vi "Initialize - Packet Page Panel.vi"(7 "Channels Listbox":refnum<vi>, 8 "error in (no error)":errorcluster, 11 "Item Ref in":T1 format="%.0x") -> (0 "error out":errorcluster, 3 "Item Ref out":T1 format="%.0x")   [LabVIEW 2019, in "UDP-Custom-Device System Explorer.lvlib"]
doc: "Initialize the Rx Channels Section Page Panel."
uses:
  UDP-Custom-Device System Explorer.lvlib
  <vilib>/NI VeriStand/Custom Device API/Custom Device Item Ref.ctl
  <vilib>/Utility/miscctls.llb/LVRowAndColumnUnsignedTypeDef.ctl
  Property Accessors/Tx Packet Accessors.lvlib
  Shared/UDP-Custom-Device Shared.lvlib
  Property Accessors/Shared Packet Accessors.lvlib
  <vilib>/NI VeriStand/Custom Device API/Custom Device API.lvlib
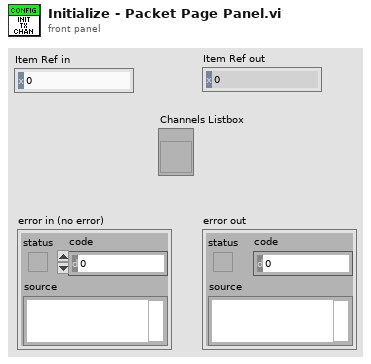
[diagram p1: front panel]
types:
  T1 = typedef "Custom Device API.lvlib/Custom Device Item Ref.ctl" = u64
  T2 = typedef "LVRowAndColumnUnsignedTypeDef.ctl" = cluster{"Row":u32, "Column":u32}
  T3 = typedef "UDP-Custom-Device Shared.lvlib/Shared - Channel Data Type.ctl" = enum16{"Boolean", "Single", "Double", "I8", "I16", "I32", "I64", "U8", "U16", "U32", "U64"}
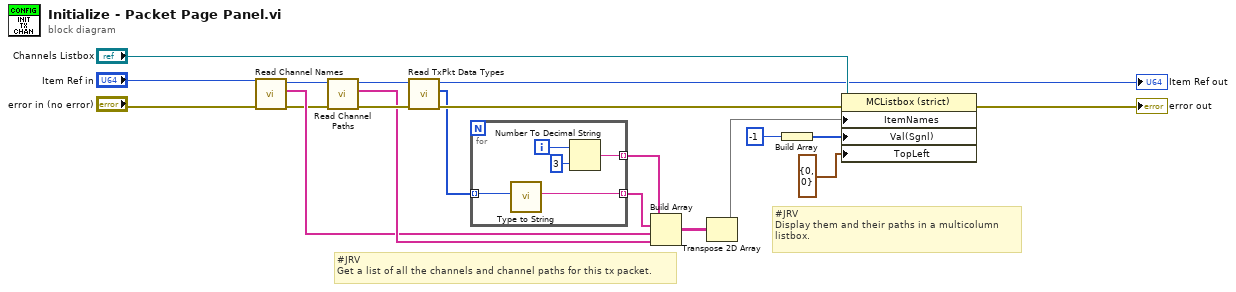
[diagram p0: block diagram]
diagram:
  # "#JRV\nDisplay them and their paths in a multicolumn\nlistbox."
  # "#JRV\nGet a list of all the channels and channel paths for this tx packet."
  n1 = call "Read Channel Names.vi"("error in (no error)"="error in (no error)", "Node Ptr"="Item Ref in") -> ("error out"=w1:errorcluster, "Channel Names"=w2:string[], "Node Ptr out"=w4:T1)  [unwired: 7 in]
  n2 = call "Read Channel Paths.vi"("error in (no error)"=w1, "Node Ptr"=w4) -> ("error out"=w7:errorcluster, "Channel Paths"=w6:string[], "Node Ptr out"=w8:T1)  [unwired: 7 in]
  n3 = call "Read TxPkt Data Types.vi"("error in (no error)"=w7, "Node Ptr"=w8) -> ("error out"=w10:errorcluster, "Data types"=w9:T3[], "Node Ptr out"=→"Item Ref out":T1)  [unwired: 7 in]
  n4 = for {
    tunnel: [w21] -> w13 mode=indexing
    tunnel: [w23] -> w12 mode=indexing
    tunnel: w9 -> [w22] mode=indexing
    i -> [w25]
    n5 = call "Type to String.vi"("Data Type"=w22) -> ("String Type"=w21:string)  [unwired: 10 in]
    n6 = Number To Decimal String(number=w25, width (-)=i16 3) -> (decimal integer string=w23:string)
  }
  n7 = Build Array(w12, w13, w2, w6) -> (w16:string[][])
  n8 = Transpose 2D Array(2D array=w16) -> (transposed array=w18:string[][])
  n9 = Build Array(-1) -> (w19:i32[])
  n10 = property class="MCListbox (strict)"(reference="Channels Listbox", error in=w10, "ItemNames"=w18, "Val(Sgnl)"=w19, "TopLeft"=T2 {"Row"=0, "Column"=0} ("Top Left Visible Cell")) -> (error out=→"error out":errorcluster)  [unwired: 1 out]
